vi "DynamicPersonality.vi"(7 "Pinned":T1={"Attc"="Auto", "Strk"="Auto", "Def"="Auto"}, 9 "Qtd Min p/ Stk":dbl=2.0, 10 "our_goalie_id":dbl, 11 "input cluster":T3={"our_robots"=[], "enemy_robots"=[], "balls"=[], "geometry"={"line_width"=0, "field_length"=0, "field_width"=0, "boundary_width"=0, "referee_width"=0, "goal_width"=0, "goal_depth"=0, "goal_wall_width"=0, "center_circle_radius"=0, "defense_radius"=0, "defense_stretch"=0, "free_kick_from_defense_dist"=0, "penalty_spot_from_field_line_dist"=0, "penalty_line_from_spot_dist"=0}, "IA Judge"={"stage"="", "command"="", "our_goalie_id"=0.0, "enemy_goalie_id"=0.0, "command enum"=enum."Halt", "Time"=enum."Azul"}, "Received Timestamp"=timestamp(0 s since 1904-01-01), "Events"={"Touch"=FALSE, "Ball out"=FALSE, "id touch"=0.0, "Ball out of \nVision"=FALSE, "Ball inside \nGoalie area"=FALSE, "Robot not responding"=FALSE, "Robots responding status"=[1.0, 1.0, 1.0, 1.0, 1.0, 1.0], "Enemy Ball \nPossession"=FALSE, "Pass State"=FALSE, "id end of pass"=0.0, "Kick"=FALSE, "Id ini Possession"=0.0, "Ball Possesion"=FALSE, "Id Possesion"=0.0}}) -> (2 "output cluster":T3={"our_robots"=[], "enemy_robots"=[], "balls"=[], "geometry"={"line_width"=0, "field_length"=0, "field_width"=0, "boundary_width"=0, "referee_width"=0, "goal_width"=0, "goal_depth"=0, "goal_wall_width"=0, "center_circle_radius"=0, "defense_radius"=0, "defense_stretch"=0, "free_kick_from_defense_dist"=0, "penalty_spot_from_field_line_dist"=0, "penalty_line_from_spot_dist"=0}, "IA Judge"={"stage"="", "command"="", "our_goalie_id"=0.0, "enemy_goalie_id"=0.0, "command enum"=enum."Halt", "Time"=enum."Azul"}, "Received Timestamp"=timestamp(0 s since 1904-01-01), "Events"={"Touch"=FALSE, "Ball out"=FALSE, "id touch"=0.0, "Ball out of \nVision"=FALSE, "Ball inside \nGoalie area"=FALSE, "Robot not responding"=FALSE, "Robots responding status"=[1.0, 1.0, 1.0, 1.0, 1.0, 1.0], "Enemy Ball \nPossession"=FALSE, "Pass State"=FALSE, "id end of pass"=0.0, "Kick"=FALSE, "Id ini Possession"=0.0, "Ball Possesion"=FALSE, "Id Possesion"=0.0}})   [LabVIEW 2017]
uses:
  Core/AI Input.ctl
  Core/AI Robot.ctl
  Intel/Functions Enum.ctl
  Intel/AttackerStates.ctl
  Core/AI Ball.ctl
  Core/Field Size.ctl
  Core/AI Judge.ctl
  Intel/Command Enum.ctl
  Util/Events/Events.ctl
  Select Personalitys.ctl
  Util/Select Auto None or Robot.ctl
panel:
  out "Dfdr\nPinned?":bool
  out "Strk\nPinned?":bool
  out "Attck\nPinned?":bool
  in  "Ids validos":u32[](array[numeric])=[42, 42, 42, 42, 42, 42, 42]
  out "Maior prioridade de \natacante é o mais\nproximo da bola?":bool
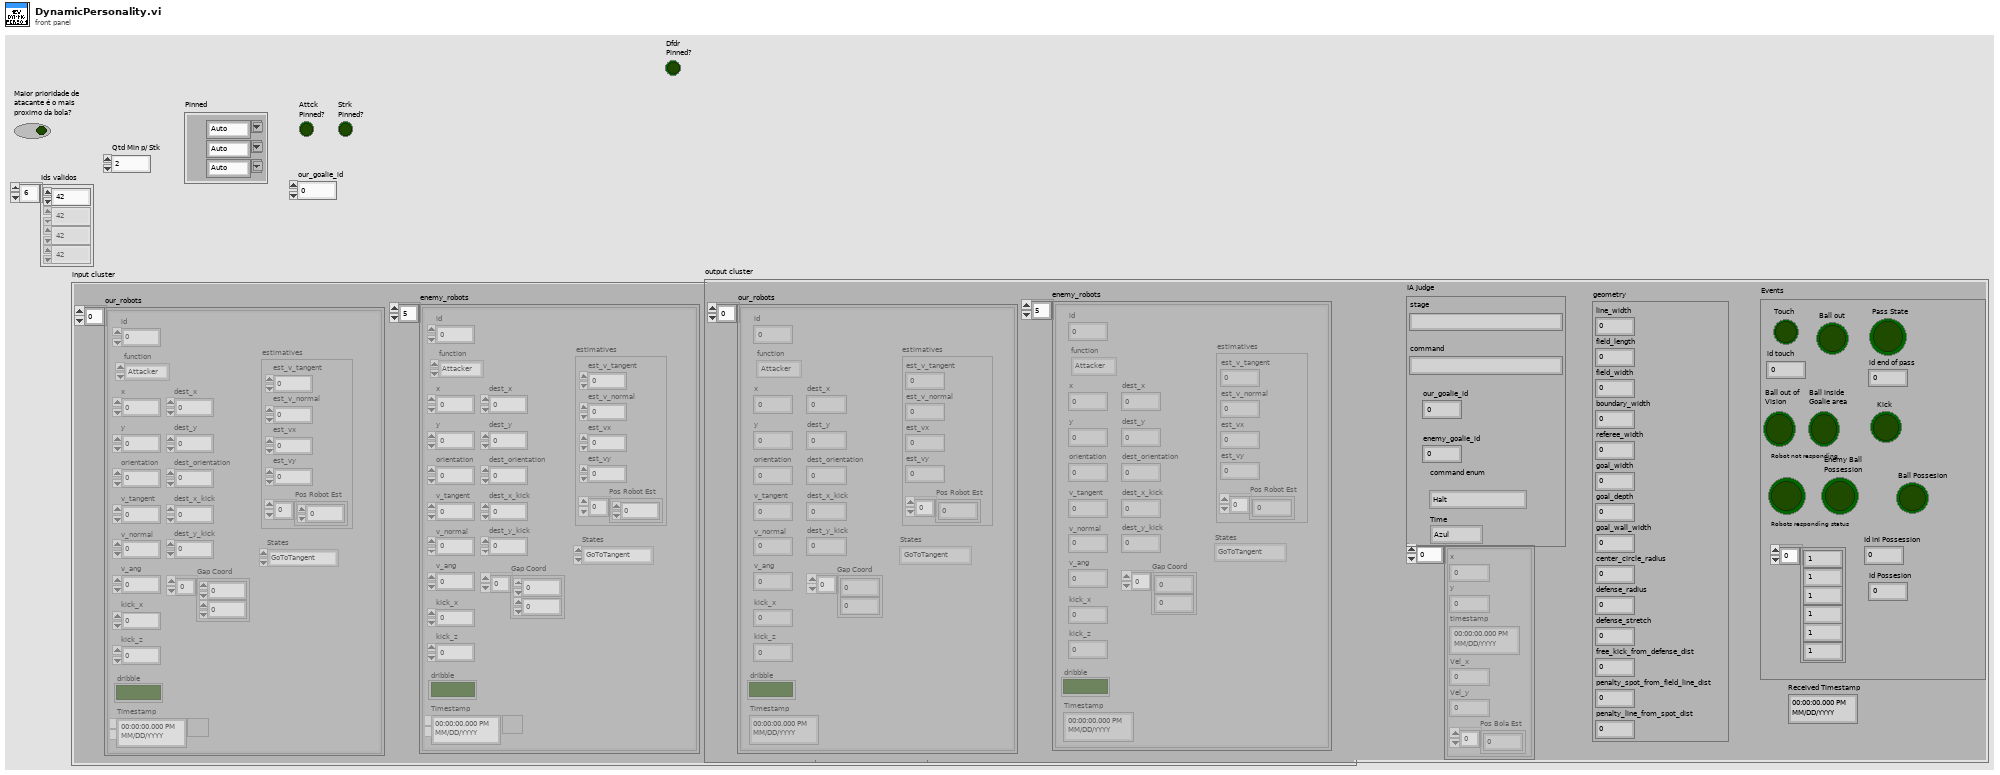
[diagram p1: front panel]
types:
  T1 = typedef "Select Personalitys.ctl" = cluster{"Attc":T2, "Strk":T2, "Def":T2}
  T2 = typedef "Select Auto None or Robot.ctl" = string
  T3 = typedef "AI Input.ctl" = cluster{"our_robots":T4[], "enemy_robots":T4[], "balls":T7[], "geometry":T8, "IA Judge":T9, "Received Timestamp":timestamp, "Events":T11}
  T4 = typedef "AI Robot.ctl" = cluster{"id":u32, "function":T5, "x":dbl, "y":dbl, "orientation":dbl, "v_tangent":dbl, "v_normal":dbl, "v_ang":dbl, "kick_x":dbl, "kick_z":dbl, "dribble":bool, "Timestamp":timestamp, "dest_x":dbl, "dest_y":dbl, "dest_orientation":dbl, "estimatives":cluster{"est_v_tangent":dbl, "est_v_normal":dbl, "est_vx":dbl, "est_vy":dbl, "Pos Robot Est":dbl[]}, "dest_x_kick":dbl, "dest_y_kick":dbl, "Gap Coord":dbl[], "States":T6}
  T5 = typedef "Functions Enum.ctl" = enum16{"Attacker", "Goalie", "Defender", "Striker", "Goto 0", "Dummy", "Kicker", "ZigZag"}
  T6 = typedef "AttackerStates.ctl" = enum16{"Pass", "GoToTangent", "BallGetting", "GoToKick", ""}
  T7 = typedef "AI Ball.ctl" = cluster{"x":dbl, "y":dbl, "timestamp":timestamp, "Vel_x":dbl, "Vel_y":dbl, "Pos Bola Est":dbl[]}
  T8 = typedef "Field Size.ctl" = cluster{"line_width":u32, "field_length":u32, "field_width":u32, "boundary_width":u32, "referee_width":u32, "goal_width":u32, "goal_depth":u32, "goal_wall_width":u32, "center_circle_radius":u32, "defense_radius":u32, "defense_stretch":u32, "free_kick_from_defense_dist":u32, "penalty_spot_from_field_line_dist":u32, "penalty_line_from_spot_dist":u32}
  T9 = typedef "AI Judge.ctl" = cluster{"stage":string, "command":string, "our_goalie_id":dbl, "enemy_goalie_id":dbl, "command enum":T10, "Time":enum16{"Azul", "Amarelo"}}
  T10 = typedef "Command Enum.ctl" = enum16{"Halt", "Stop", "Force Start", "PKA Normal Start", "Prepare Kickoff Ally", "PKE Normal Start", "Prepare Kickoff Enemy", "Prepare Penalty Ally", "PPA Normal Start", "Prepare Penalty Enemy", "PPE Normal Start", "Direct Free Enemy", "Direct Free Ally", "Indirect Free Enemy", "Indirect Free Ally", "Timeout Enemy", "Timeout Ally", "Goal Enemy", "Goal Ally", "Ball Placement Enemy", "Ball Placement Ally", "Normal Half Time", "Extra Time Break", "Extra Half Time", "None", "Post Game"}
  T11 = typedef "Events.ctl" = cluster{"Touch":bool, "Ball out":bool, "id touch":dbl, "Ball out of \nVision":bool, "Ball inside \nGoalie area":bool, "Robot not responding":bool, "Robots responding status":dbl[], "Enemy Ball \nPossession":bool, "Pass State":bool, "id end of pass":dbl, "Kick":bool, "Id ini Possession":dbl, "Ball Possesion":bool, "Id Possesion":dbl}
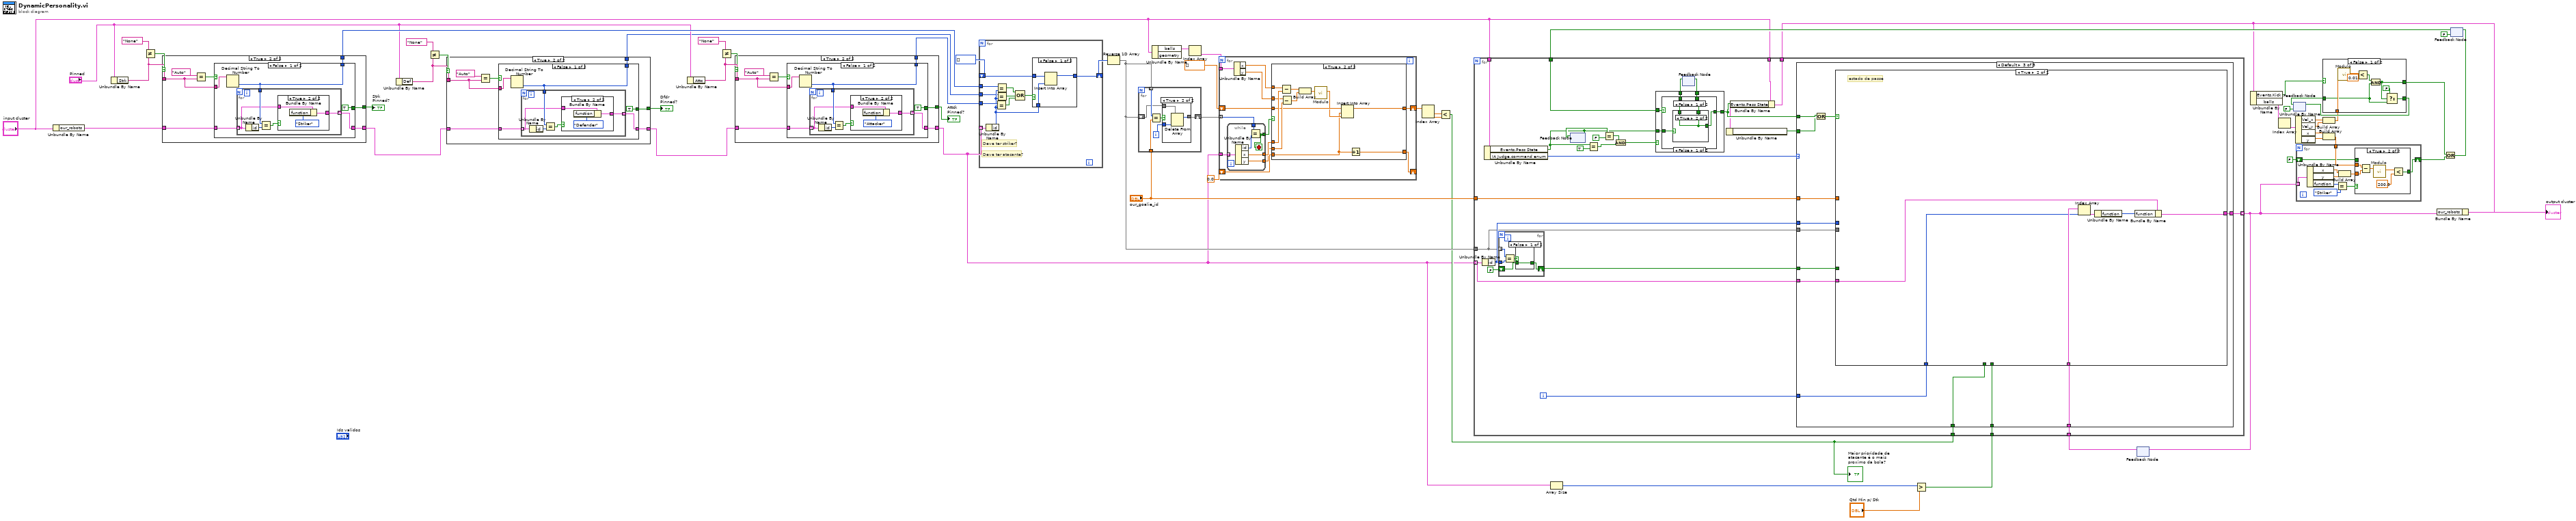
[diagram p0: block diagram]
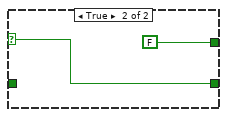
[diagram p2: hidden frame]
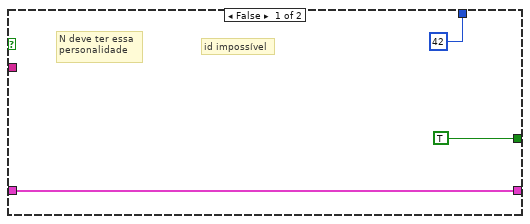
[diagram p4: hidden frame]
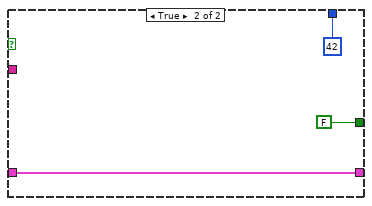
[diagram p6: hidden frame]
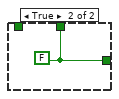
[diagram p10: hidden frame]
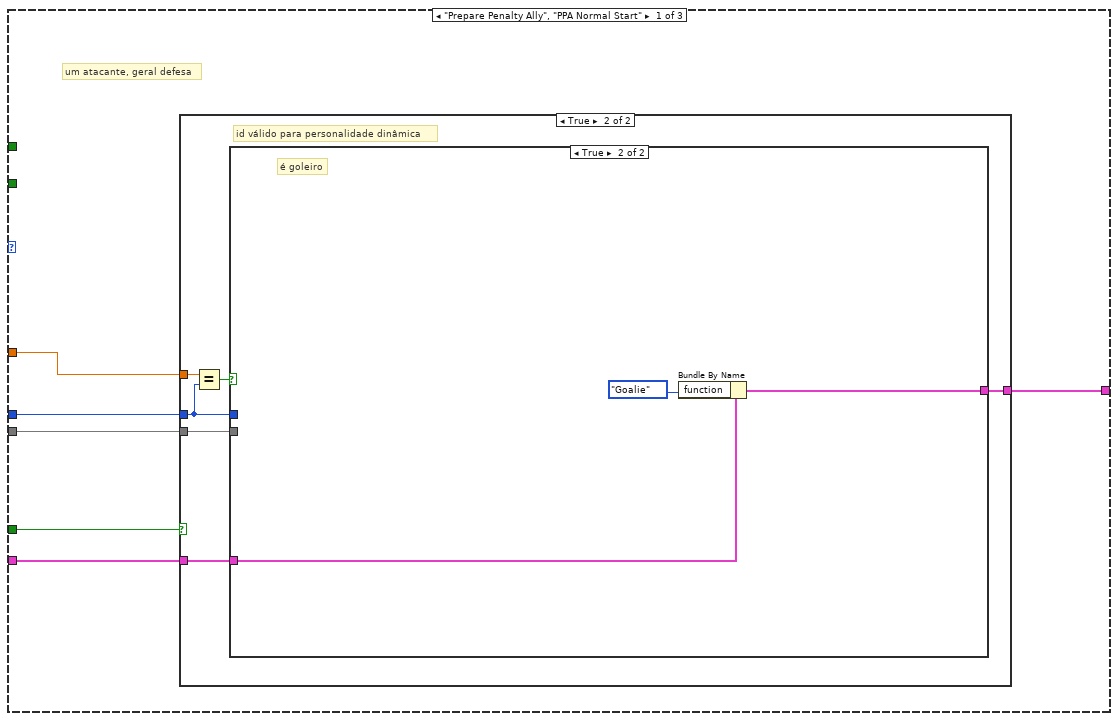
[diagram p12: hidden frame]
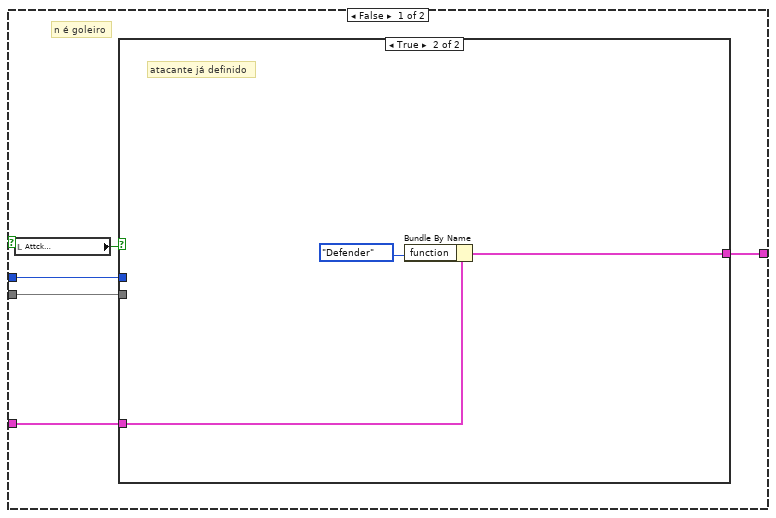
[diagram p14: hidden frame]
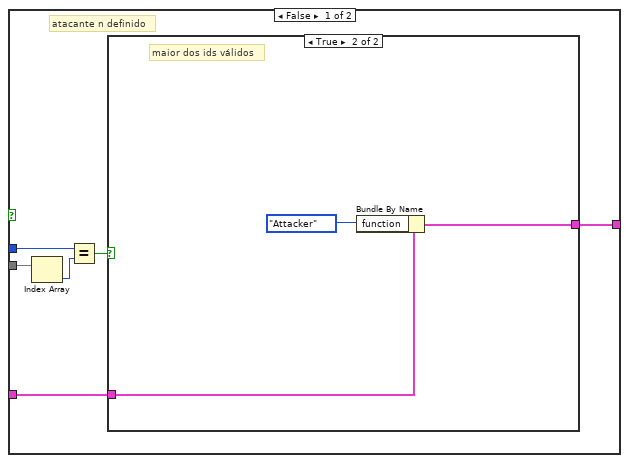
[diagram p15: hidden frame]
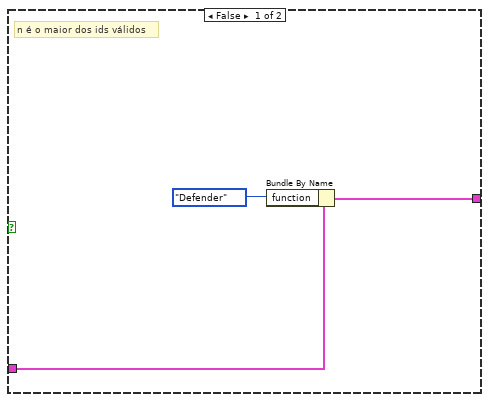
[diagram p16: hidden frame]
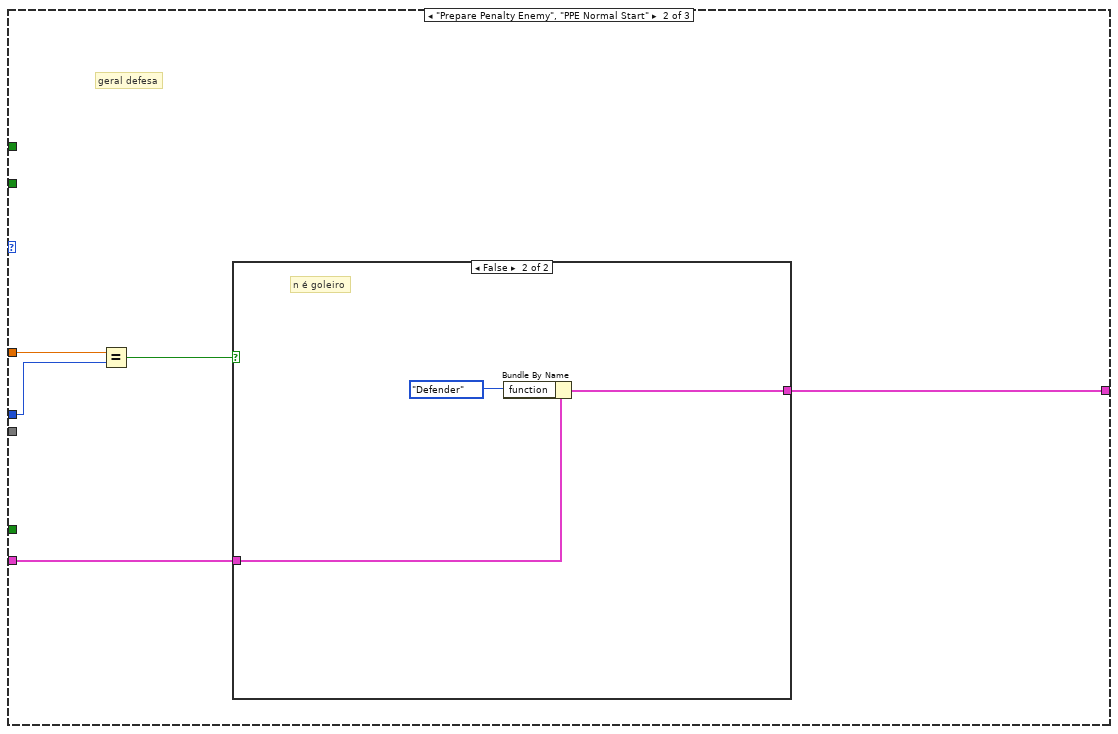
[diagram p17: hidden frame]
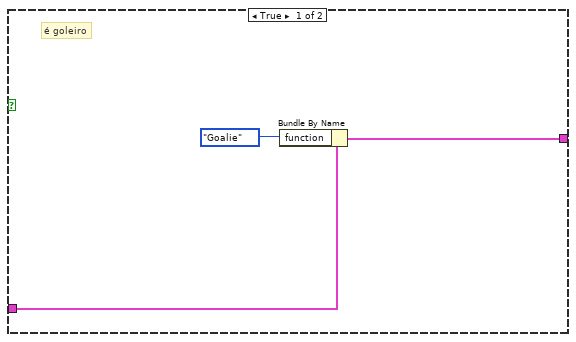
[diagram p18: hidden frame]
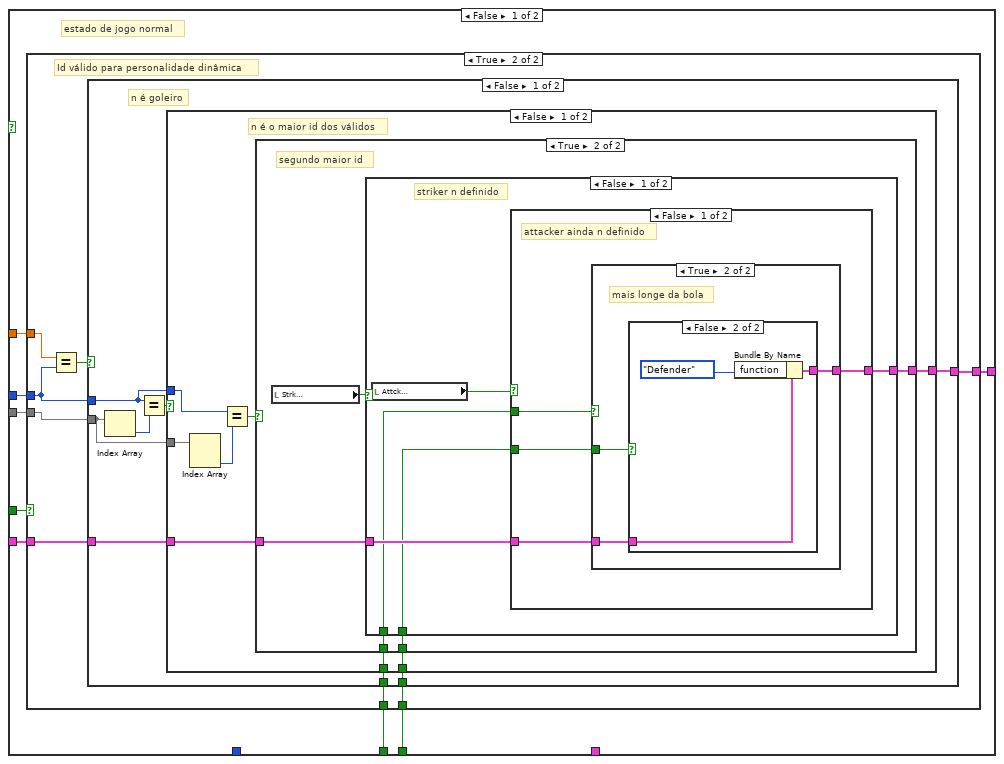
[diagram p19: hidden frame]
diagram:
  n1 = Unbundle By Name("input cluster") -> ("our_robots"=w56:T4[])
  n2 = Unbundle By Name("Pinned") -> ("Strk"=w57:T2)
  n3 = Not Equal?(x=T2 "None", y=w57) -> (x != y?=w58:bool)
  n4 = case shown="True" w58 {
    tunnel: w57 -> [_ w67]
    tunnel: w56 -> [w62 w66]
    tunnel: [w62 w65] -> w28
    tunnel: [TRUE w64] -> w34
    tunnel: [u32 42 ("Id Maior\nprioridade\natacante") w63] -> w51
    frame False {
      # "id impossível"
      # "N deve ter essa \npersonalidade"
    }
    frame True {
      n5 = Equal?(x=T2 "Auto", y=w67) -> (x = y?=w68:bool)
      n6 = case shown="False" w68 {
        tunnel: w67 -> [w74 _]
        tunnel: w66 -> [w73 w86]
        tunnel: [w72 w86] -> w65
        tunnel: [TRUE FALSE] -> w64
        tunnel: [w70 42] -> w63
        frame False {
          n7 = Decimal String To Number(string=w74) -> (number=w70:i32)  [unwired: 2 in, 1 out]
          n8 = for {
            tunnel: w73 -> [w77] mode=indexing
            tunnel: w70 -> [w78]
            tunnel: [w76] -> w72 mode=indexing
            n9 = Unbundle By Name(w77) -> ("id"=w79:u32)
            n10 = Equal?(x=w78, y=w79) -> (x = y?=w75:bool)
            n11 = case shown="True" w75 {
              tunnel: w77 -> [w80 w83]
              tunnel: [w80 w82] -> w76
              frame False {
              }
              frame True {
                n12 = Bundle By Name(cluster=w83, "function"=Functions_Enum."Striker") -> (w82:T4)
              }
            }
          }
        }
        frame True {
        }
      }
    }
  }
  "Strk\nPinned?" <- w34
  n13 = Unbundle By Name("Pinned") -> ("Def"=w30:T2)
  n14 = Not Equal?(x=T2 "None", y=w30) -> (x != y?=w31:bool)
  n15 = case shown="True" w31 {
    tunnel: w30 -> [_ w94]
    tunnel: w28 -> [w89 w93]
    tunnel: [w89 w92] -> w27
    tunnel: [TRUE w91] -> w29
    tunnel: [u32 42 ("Id Maior\nprioridade\natacante") w90] -> w25
    frame False {
      # "id impossível"
      # "N deve ter essa \npersonalidade"
    }
    frame True {
      n16 = Equal?(x=T2 "Auto", y=w94) -> (x = y?=w95:bool)
      n17 = case shown="False" w95 {
        tunnel: w94 -> [w101 _]
        tunnel: w93 -> [w100 w113]
        tunnel: [w99 w113] -> w92
        tunnel: [TRUE FALSE] -> w91
        tunnel: [w97 42] -> w90
        frame False {
          n18 = Decimal String To Number(string=w101) -> (number=w97:i32)  [unwired: 2 in, 1 out]
          n19 = for {
            tunnel: w100 -> [w104] mode=indexing
            tunnel: w97 -> [w105]
            tunnel: [w103] -> w99 mode=indexing
            n20 = Unbundle By Name(w104) -> ("id"=w106:u32)
            n21 = Equal?(x=w105, y=w106) -> (x = y?=w102:bool)
            n22 = case shown="True" w102 {
              tunnel: w104 -> [w107 w110]
              tunnel: [w107 w109] -> w103
              frame False {
              }
              frame True {
                n23 = Bundle By Name(cluster=w110, "function"=Functions_Enum."Defender") -> (w109:T4)
              }
            }
          }
        }
        frame True {
        }
      }
    }
  }
  "Dfdr\nPinned?" <- w29
  n24 = Unbundle By Name("Pinned") -> ("Attc"=w54:T2)
  n25 = Not Equal?(x=T2 "None", y=w54) -> (x != y?=w53:bool)
  n26 = case shown="True" w53 {
    tunnel: w54 -> [_ w121]
    tunnel: w27 -> [w116 w120]
    tunnel: [w116 w119] -> w24
    tunnel: [TRUE w118] -> w33
    tunnel: [42 w117] -> w52
    frame False {
      (unwired) u32 42 ("Id Maior\nprioridade\natacante")
      # "id impossível"
      # "N deve ter essa \npersonalidade"
    }
    frame True {
      n27 = Equal?(x=T2 "Auto", y=w121) -> (x = y?=w122:bool)
      n28 = case shown="False" w122 {
        tunnel: w121 -> [w128 _]
        tunnel: w120 -> [w127 w140]
        tunnel: [w126 w140] -> w119
        tunnel: [TRUE FALSE] -> w118
        tunnel: [w124 42] -> w117
        frame False {
          n29 = Decimal String To Number(string=w128) -> (number=w124:i32)  [unwired: 2 in, 1 out]
          n30 = for {
            tunnel: w127 -> [w131] mode=indexing
            tunnel: w124 -> [w132]
            tunnel: [w130] -> w126 mode=indexing
            n31 = Unbundle By Name(w131) -> ("id"=w133:u32)
            n32 = Equal?(x=w132, y=w133) -> (x = y?=w129:bool)
            n33 = case shown="True" w129 {
              tunnel: w131 -> [w134 w137]
              tunnel: [w134 w136] -> w130
              frame False {
              }
              frame True {
                n34 = Bundle By Name(cluster=w137, "function"=Functions_Enum."Attacker") -> (w136:T4)
              }
            }
          }
        }
        frame True {
        }
      }
    }
  }
  "Attck\nPinned?" <- w33
  n35 = for {
    tunnel: w24 -> [w151] mode=indexing
    tunnel: w52 -> [w150]
    shift-right: [w146] -> w49
    shift-left: u32[] [] -> [w147]
    tunnel: w51 -> [w149]
    tunnel: w25 -> [w143]
    # "Deve ter striker?"
    # "Deve ter atacante?"
    n36 = Unbundle By Name(w151) -> ("id"=w144:u32)
    n37 = Equal?(x=w150, y=w144) -> (x = y?=w148:bool)
    n38 = Equal?(x=w149, y=w144) -> (x = y?=w142:bool)
    n39 = Equal?(x=w143, y=w144) -> (x = y?=w141:bool)
    n40 = Compound Arithmetic op=OR(w142, w141, w148) -> (w145:bool)
    n41 = case shown="False" w145 {
      tunnel: [w152 w155] -> w146
      tunnel: w147 -> [w154 w155]
      tunnel: w144 -> [w153 _]
      frame False {
        n42 = Insert Into Array(array=w154, new element=w153) -> (w152:u32[])  [unwired: 1 in]
      }
      frame True {
      }
    }
  }
  n43 = Reverse 1D Array(array=w49) -> (reversed array=w46:u32[])
  n44 = for {
    tunnel: w46 -> [w160] mode=indexing
    tunnel: "our_goalie_id" -> [w159]
    shift-right: [w156] -> w43
    shift-left: w46 -> [w158]
    i -> [w157]
    n45 = Equal?(x=w160, y=w159) -> (x = y?=w161:bool)
    n46 = case shown="True" w161 {
      tunnel: w158 -> [w162 w165]
      tunnel: w157 -> [_ w164]
      tunnel: [w162 w163] -> w156
      frame False {
      }
      frame True {
        n47 = Delete From Array(array=w165, index=w164) -> (array with subset deleted=w163:u32[])  [unwired: 1 in, 1 out]
      }
    }
  }
  n48 = Unbundle By Name("input cluster") -> ("balls"=w45:T7[])  [unwired: 1 out]
  n49 = Index Array(array=w45) -> (element=w44:T7)  [unwired: 1 in]
  n50 = for {
    tunnel: w44 -> [w174]
    tunnel: w43 -> [w167] mode=indexing
    tunnel: w24 -> [w177]
    shift-right: [w171] -> w41
    shift-left: dbl[] [] -> [w170]
    shift-right: [w168] -> _
    shift-left: 0.0 -> [w169]
    n51 = while {
      tunnel: w177 -> [w183] mode=indexing
      tunnel: [w182] -> w176
      tunnel: [w181] -> w175
      tunnel: w167 -> [w180]
      tunnel: [w178] -> w166
      stop <- w178 stop-if-true
      n52 = Unbundle By Name(w183) -> ("id"=w179:u32, "x"=w182:dbl, "y"=w181:dbl)
      n53 = Equal?(x=w180, y=w179) -> (x = y?=w178:bool)
    }
    n54 = Unbundle By Name(w174) -> ("x"=w173:dbl, "y"=w172:dbl)
    n55 = case shown="True" w166 {
      tunnel: w176 -> [_ w196]
      tunnel: w175 -> [_ w194]
      tunnel: w173 -> [_ w197]
      tunnel: w172 -> [_ w195]
      tunnel: [w185 w190] -> w171
      tunnel: w170 -> [w185 w189]
      tunnel: w169 -> [w184 w187]
      tunnel: [w184 w186] -> w168
      frame False {
      }
      frame True {
        n56 = Subtract(x=w197, y=w196) -> (x-y=w193:dbl)
        n57 = Subtract(x=w195, y=w194) -> (x-y=w192:dbl)
        n58 = Build Array(w193, w192) -> (w191:dbl[])
        n59 = call "Modulo.vi"("2D vector"=w191) -> ("Modulo"=w188:dbl)  [unwired: 10 in]
        n60 = Insert Into Array(array=w189, index=w187, new element=w188) -> (w190:dbl[])
        n61 = Increment(x=w187) -> (x+1=w186:dbl)
      }
    }
  }
  n62 = Index Array(array=w41) -> (element #1=w39:dbl, element #2=w40:dbl)  [unwired: 2 in]
  n63 = Less?(x=w39, y=w40) -> (x < y?=w38:bool)
  "Maior prioridade de \natacante é o mais\nproximo da bola?" <- w38
  n64 = Array Size(array=w24) -> (size(s)=w36:i32)
  n65 = Greater?(x=w36, y="Qtd Min p/ Stk") -> (0:w37:bool)
  n66 = feedback #1() -> (w23:T4[])  [unwired: 1 in]
  n67 = feedback #2(FALSE ("Kick")) -> (w7:bool)
  n68 = feedback #3(FALSE) -> (w15:bool)
  n69 = for {
    tunnel: w24 -> [w214] mode=indexing
    tunnel: w46 -> [w220]
    tunnel: "our_goalie_id" -> [w222]
    tunnel: [w221] -> w22 mode=indexing
    tunnel: w38 -> [w218]
    tunnel: w37 -> [w217]
    tunnel: "input cluster" -> [w216]
    tunnel: w23 -> [w213]
    tunnel: w15 -> [w209]
    tunnel: "input cluster" -> [w201]
    tunnel: [w199] -> w12
    i -> [w212]
    n70 = Unbundle By Name(w214) -> ("id"=w223:u32)
    n71 = Unbundle By Name(w216) -> ("Events.Pass State"=w207:bool, "IA Judge.command enum"=w215:T10)
    n72 = for {
      tunnel: w220 -> [w434] mode=indexing
      tunnel: w223 -> [w435]
      shift-right: [w432] -> w219
      shift-left: FALSE -> [w433]
      n73 = Equal?(x=w434, y=w435) -> (x = y?=w431:bool)
      n74 = case shown="False" w431 {
        tunnel: w433 -> [w436 _]
        tunnel: [w436 TRUE] -> w432
        frame False {
        }
        frame True {
        }
      }
    }
    n75 = feedback-in #4(w207) -> ()
    n76 = feedback #4() -> (w208:bool)  [unwired: 1 in]
    n77 = Equal?(x=w207, y=TRUE) -> (x = y?=w203:bool)
    n78 = Equal?(x=w208, y=FALSE) -> (x = y?=w204:bool)
    n79 = And(x=w204, y=w203) -> (x .and. y?=w202:bool)
    n80 = feedback #5() -> (w210:bool)  [unwired: 1 in]
    n81 = case shown="False" w202 {
      selector: w202 -> [_ w237]
      tunnel: [w229 w237] -> w211
      tunnel: w210 -> [w228 _]
      tunnel: w209 -> [w227 _]
      tunnel: [w226 w237] -> w200
      tunnel: w207 -> [w225 _]
      frame False {
        n82 = case shown="False" w227 {
          tunnel: w225 -> [w233 _]
          tunnel: [w230 w236] -> w229
          tunnel: w228 -> [w232 _]
          tunnel: [w231 w236] -> w226
          frame False {
            n83 = case shown="True" w233 {
              selector: w233 -> [w234 _]
              tunnel: w232 -> [_ w235]
              tunnel: [w234 w235] -> w231
              tunnel: [w234 w235] -> w230
              frame False {
              }
              frame True {
              }
            }
          }
          frame True {
            w236 = FALSE
          }
        }
      }
      frame True {
      }
    }
    n84 = feedback-in #5(w211) -> ()
    n85 = Bundle By Name(cluster=w201, "Events.Pass State"=w200) -> (w199:T3)
    n86 = Unbundle By Name(w199) -> ("Events.Ball out of \nVision"=w198:bool)
    n87 = case shown="Default" w215 {
      tunnel: w223 -> [w240 w274 w297]
      tunnel: w222 -> [w238 w275 w296]
      tunnel: w214 -> [w242 w278 w295]
      tunnel: [w243 w277 w294] -> w221
      tunnel: w220 -> [w239 _ w293]
      tunnel: w219 -> [w241 _ w292]
      tunnel: w218 -> [_ _ w291]
      tunnel: w217 -> [_ _ w290]
      tunnel: w213 -> [_ _ w289]
      tunnel: w212 -> [_ _ w288]
      tunnel: w200 -> [_ _ w286]
      tunnel: w198 -> [_ _ w285]
      frame "Prepare Penalty Ally", "PPA Normal Start" {
        # "um atacante, geral defesa"
        n88 = case shown="True" w241 {
          tunnel: [w244 w250] -> w243
          tunnel: w242 -> [w244 w249]
          tunnel: w240 -> [_ w246]
          tunnel: w239 -> [_ w248]
          tunnel: w238 -> [_ w245]
          frame False {
            # "personalidade já definida"
          }
          frame True {
            # "id válido para personalidade dinâmica"
            n89 = Equal?(x=w245, y=w246) -> (x = y?=w247:bool)
            n90 = case shown="True" w247 {
              tunnel: [w255 w272] -> w250
              tunnel: w249 -> [w254 w271]
              tunnel: w246 -> [w252 _]
              tunnel: w248 -> [w251 _]
              frame False {
                # "n é goleiro"
                n91 = local read "Attck\nPinned?"() -> (w253:bool)
                n92 = case shown="True" w253 {
                  tunnel: [w261 w269] -> w255
                  tunnel: w254 -> [w260 w268]
                  tunnel: w252 -> [w258 _]
                  tunnel: w251 -> [w256 _]
                  frame False {
                    # "atacante n definido"
                    n93 = Index Array(array=w256) -> (element=w257:u32)  [unwired: 1 in]
                    n94 = Equal?(x=w258, y=w257) -> (x = y?=w259:bool)
                    n95 = case shown="True" w259 {
                      tunnel: [w263 w266] -> w261
                      tunnel: w260 -> [w262 w265]
                      frame False {
                        # "n é o maior dos ids válidos"
                        n96 = Bundle By Name(cluster=w262, "function"=Functions_Enum."Defender") -> (w263:T4)
                      }
                      frame True {
                        # "maior dos ids válidos"
                        n97 = Bundle By Name(cluster=w265, "function"=Functions_Enum."Attacker") -> (w266:T4)
                      }
                    }
                  }
                  frame True {
                    # "atacante já definido"
                    n98 = Bundle By Name(cluster=w268, "function"=Functions_Enum."Defender") -> (w269:T4)
                  }
                }
              }
              frame True {
                # "é goleiro"
                n99 = Bundle By Name(cluster=w271, "function"=Functions_Enum."Goalie") -> (w272:T4)
              }
            }
          }
        }
      }
      frame "Prepare Penalty Enemy", "PPE Normal Start" {
        # "geral defesa"
        n100 = Equal?(x=w275, y=w274) -> (x = y?=w276:bool)
        n101 = case shown="False" w276 {
          tunnel: w278 -> [w281 w284]
          tunnel: [w280 w283] -> w277
          frame True {
            # "é goleiro"
            n102 = Bundle By Name(cluster=w281, "function"=Functions_Enum."Goalie") -> (w280:T4)
          }
          frame False {
            # "n é goleiro"
            n103 = Bundle By Name(cluster=w284, "function"=Functions_Enum."Defender") -> (w283:T4)
          }
        }
      }
      frame Default {
        n104 = Or(x=w286, y=w285) -> (x .or. y?=w287:bool)
        n105 = case shown="True" w287 {
          tunnel: w297 -> [w305 _]
          tunnel: w296 -> [w304 _]
          tunnel: w295 -> [w303 w427]
          tunnel: [w302 w426] -> w294
          tunnel: w293 -> [w301 _]
          tunnel: w292 -> [w300 _]
          tunnel: w291 -> [w299 _]
          tunnel: w290 -> [w298 _]
          tunnel: w289 -> [_ w430]
          tunnel: w288 -> [_ w429]
          frame False {
            # "estado de jogo normal"
            n106 = case shown="True" w300 {
              tunnel: w305 -> [_ w310]
              tunnel: w304 -> [_ w314]
              tunnel: w303 -> [w306 w312]
              tunnel: [w306 w311] -> w302
              tunnel: w301 -> [_ w309]
              tunnel: w299 -> [_ w308]
              tunnel: w298 -> [_ w307]
              frame False {
                # "Personalidade já definida"
              }
              frame True {
                # "Id válido para personalidade dinâmica"
                n107 = Equal?(x=w314, y=w310) -> (x = y?=w313:bool)
                n108 = case shown="False" w313 {
                  tunnel: w312 -> [w319 w423]
                  tunnel: [w320 w422] -> w311
                  tunnel: w310 -> [w317 _]
                  tunnel: w309 -> [w318 _]
                  tunnel: w308 -> [w316 _]
                  tunnel: w307 -> [w315 _]
                  frame False {
                    # "n é goleiro"
                    n109 = Index Array(array=w318) -> (element=w321:u32)  [unwired: 1 in]
                    n110 = Equal?(x=w317, y=w321) -> (x = y?=w322:bool)
                    n111 = case shown="False" w322 {
                      tunnel: [w327 w381] -> w320
                      tunnel: w319 -> [w328 w380]
                      tunnel: w318 -> [w329 _]
                      tunnel: w317 -> [w326 _]
                      tunnel: w316 -> [w324 w379]
                      tunnel: w315 -> [w323 w378]
                      frame False {
                        # "n é o maior id dos válidos"
                        n112 = Index Array(array=w329) -> (element #2=w325:u32)  [unwired: 2 in, 1 out]
                        n113 = Equal?(x=w326, y=w325) -> (x = y?=w330:bool)
                        n114 = case shown="True" w330 {
                          tunnel: w328 -> [w331 w337]
                          tunnel: [w332 w336] -> w327
                          tunnel: w324 -> [_ w335]
                          tunnel: w323 -> [_ w334]
                          frame False {
                            # "n é o segundo maior id"
                            n115 = Bundle By Name(cluster=w331, "function"=Functions_Enum."Defender") -> (w332:T4)
                          }
                          frame True {
                            # "segundo maior id"
                            n116 = local read "Strk\nPinned?"() -> (w338:bool)
                            n117 = case shown="False" w338 {
                              tunnel: w337 -> [w342 w370]
                              tunnel: [w343 w369] -> w336
                              tunnel: w335 -> [w340 _]
                              tunnel: w334 -> [w339 _]
                              frame False {
                                # "striker n definido"
                                n118 = local read "Attck\nPinned?"() -> (w341:bool)
                                n119 = case shown="False" w341 {
                                tunnel: [w347 w367] -> w343
                                tunnel: w342 -> [w346 w366]
                                tunnel: w340 -> [w345 _]
                                tunnel: w339 -> [w344 _]
                                frame False {
                                # "attacker ainda n definido"
                                n120 = case shown="True" w345 {
                                tunnel: [w350 w359] -> w347
                                tunnel: w346 -> [w349 w358]
                                tunnel: w344 -> [w348 w357]
                                frame False {
                                # "mais perto da bola"
                                n121 = case shown="True" w348 {
                                tunnel: [w352 w355] -> w350
                                tunnel: w349 -> [w351 w354]
                                frame True {
                                n122 = Bundle By Name(cluster=w351, "function"=Functions_Enum."Attacker") -> (w352:T4)
                                }
                                frame False {
                                n123 = Bundle By Name(cluster=w354, "function"=Functions_Enum."Defender") -> (w355:T4)
                                }
                                }
                                }
                                frame True {
                                # "mais longe da bola"
                                n124 = case shown="False" w357 {
                                tunnel: [w361 w364] -> w359
                                tunnel: w358 -> [w360 w363]
                                frame True {
                                n125 = Bundle By Name(cluster=w360, "function"=Functions_Enum."Striker") -> (w361:T4)
                                }
                                frame False {
                                n126 = Bundle By Name(cluster=w363, "function"=Functions_Enum."Defender") -> (w364:T4)
                                }
                                }
                                }
                                }
                                }
                                frame True {
                                # "attacker travado"
                                n127 = Bundle By Name(cluster=w366, "function"=Functions_Enum."Defender") -> (w367:T4)
                                }
                                }
                              }
                              frame True {
                                # "striker travado"
                                n128 = local read "Attck\nPinned?"() -> (w371:bool)
                                n129 = case shown="False" w371 {
                                tunnel: w370 -> [w372 w375]
                                tunnel: [w373 w376] -> w369
                                frame False {
                                # "atacante n definido"
                                n130 = Bundle By Name(cluster=w372, "function"=Functions_Enum."Defender") -> (w373:T4)
                                }
                                frame True {
                                # "atacante travado"
                                n131 = Bundle By Name(cluster=w375, "function"=Functions_Enum."Defender") -> (w376:T4)
                                }
                                }
                              }
                            }
                          }
                        }
                      }
                      frame True {
                        # "maior id dos válidos"
                        n132 = local read "Attck\nPinned?"() -> (w382:bool)
                        n133 = case shown="False" w382 {
                          tunnel: [w386 w408] -> w381
                          tunnel: w380 -> [w385 w407]
                          tunnel: w379 -> [w384 _]
                          tunnel: w378 -> [w383 w406]
                          frame False {
                            # "Atacante ainda n definido"
                            n134 = case shown="False" w384 {
                              tunnel: [w390 w404] -> w386
                              tunnel: w385 -> [w389 w403]
                              tunnel: w383 -> [w387 _]
                              frame False {
                                # "n é o mais perto da bola"
                                n135 = local read "Strk\nPinned?"() -> (w388:bool)
                                n136 = case shown="False" w388 {
                                tunnel: [w393 w401] -> w390
                                tunnel: w389 -> [w392 w400]
                                tunnel: w387 -> [w391 _]
                                frame False {
                                n137 = case shown="False" w391 {
                                tunnel: [w395 w398] -> w393
                                tunnel: w392 -> [w394 w397]
                                frame True {
                                n138 = Bundle By Name(cluster=w394, "function"=Functions_Enum."Striker") -> (w395:T4)
                                }
                                frame False {
                                n139 = Bundle By Name(cluster=w397, "function"=Functions_Enum."Attacker") -> (w398:T4)
                                }
                                }
                                }
                                frame True {
                                n140 = Bundle By Name(cluster=w400, "function"=Functions_Enum."Attacker") -> (w401:T4)
                                }
                                }
                              }
                              frame True {
                                # "mais perto da bola"
                                n141 = Bundle By Name(cluster=w403, "function"=Functions_Enum."Attacker") -> (w404:T4)
                              }
                            }
                          }
                          frame True {
                            # "Atacande já travado"
                            n142 = local read "Strk\nPinned?"() -> (w409:bool)
                            n143 = case shown="True" w409 {
                              tunnel: [w412 w420] -> w408
                              tunnel: w407 -> [w411 w419]
                              tunnel: w406 -> [w410 _]
                              frame False {
                                # "Striker ainda n definido"
                                n144 = case shown="False" w410 {
                                tunnel: [w414 w417] -> w412
                                tunnel: w411 -> [w413 w416]
                                frame True {
                                n145 = Bundle By Name(cluster=w413, "function"=Functions_Enum."Striker") -> (w414:T4)
                                }
                                frame False {
                                n146 = Bundle By Name(cluster=w416, "function"=Functions_Enum."Defender") -> (w417:T4)
                                }
                                }
                              }
                              frame True {
                                # "Sobra defesa"
                                # "Striker já travado"
                                n147 = Bundle By Name(cluster=w419, "function"=Functions_Enum."Defender") -> (w420:T4)
                              }
                            }
                          }
                        }
                      }
                    }
                  }
                  frame True {
                    # "é goleiro"
                    n148 = Bundle By Name(cluster=w423, "function"=Functions_Enum."Goalie") -> (w422:T4)
                  }
                }
              }
            }
          }
          frame True {
            # "estado de passe"
            n149 = Index Array(array=w430, index=w429) -> (element=w428:T4)
            n150 = Unbundle By Name(w428) -> ("function"=w425:T5)
            n151 = Bundle By Name(cluster=w427, "function"=w425) -> (w426:T4)
          }
        }
      }
    }
  }
  n152 = feedback-in #1(w22) -> ()
  n153 = Unbundle By Name(w12) -> ("Events.Kick"=w8:bool, "balls"=w21:T7[])
  n154 = Index Array(array=w21) -> (element=w20:T7)  [unwired: 1 in]
  n155 = Unbundle By Name(w20) -> ("Vel_x"=w6:dbl, "Vel_y"=w5:dbl, "x"=w19:dbl, "y"=w18:dbl)
  n156 = Build Array(w6, w5) -> (w4:dbl[])
  n157 = case shown="False" w8 {
    selector: w8 -> [_ w447]
    tunnel: [w439 w447] -> w9
    tunnel: w7 -> [w438 _]
    tunnel: w4 -> [w445 _]
    tunnel: [w441 FALSE] -> w1
    frame False {
      n158 = call "Modulo.vi"("2D vector"=w445) -> ("Modulo"=w444:dbl)  [unwired: 10 in]
      n159 = Less?(x=w444, y=0.01) -> (x < y?=w442:bool)
      n160 = And(x=w442, y=w438) -> (x .and. y?=w441:bool)
      n161 = Select(t=FALSE ("Kick"), s=w441, f=w438) -> (s? t:f=w439:bool)
    }
    frame True {
    }
  }
  n162 = feedback-in #2(w9) -> ()
  n163 = Build Array(w19, w18) -> (w17:dbl[])
  n164 = for {
    tunnel: w22 -> [w457] mode=indexing
    tunnel: w17 -> [w450]
    shift-right: [w449] -> w3
    shift-left: FALSE -> [w448]
    n165 = Unbundle By Name(w457) -> ("x"=w453:dbl, "y"=w452:dbl, "function"=w456:T5)
    n166 = Equal?(x=w456, y=Functions_Enum."Striker") -> (x = y?=w454:bool)
    n167 = Build Array(w453, w452) -> (w451:dbl[])
    n168 = case shown="True" w454 {
      tunnel: w451 -> [_ w463]
      tunnel: w450 -> [_ w464]
      tunnel: [w458 w459] -> w449
      tunnel: w448 -> [w458 _]
      frame False {
      }
      frame True {
        n169 = Subtract(x=w464, y=w463) -> (x-y=w462:dbl[])
        n170 = call "Modulo.vi"("2D vector"=w462) -> ("Modulo"=w461:dbl)  [unwired: 10 in]
        n171 = Less?(x=w461, y=200.0) -> (x < y?=w459:bool)
      }
    }
  }
  n172 = Bundle By Name(cluster=w12, "our_robots"=w22) -> (→"output cluster":T3)
  n173 = Or(x=w1, y=w3) -> (x .or. y?=w2:bool)
  n174 = feedback-in #3(w2) -> ()
